vi "Pat 3.0.vi"(8 "error in":errorcluster, 11 "Father of all uServices in":refnum<class "Father of all uServices.lvclass">) -> (0 "error out":errorcluster, 3 "Father of all uServices out":refnum<class "Father of all uServices.lvclass">)   [LabVIEW 2026, in "TALOS.lvlib" / "Father of all uServices.lvlib" / "Father of all uServices.lvclass"]
uses:
  Father of all uServices.lvclass
  C:/LabVIEW Code/TALOS/talos/Ancestor/Ancestor/Ancestor.lvclass
  Ancestor/Ancestor/Ancestor.lvclass/Ancestor.ctl
  Classes/uService List/uService List.lvclass/uService List.ctl
  Classes/uService List/Set Last Pat.vi
  Classes/uService List/Set Online Status.vi
  Ancestor/Ancestor/Read ID.vi
  Ancestor/Ancestor/Write uS List Ref.vi
  Support VIs/Generate Error.vi
  FGV/Error Memory/Get Error Description.vi
  Support VIs/Get PC name.vi
  Support VIs/Get Class Name.vi
  <vilib>/Utility/error.llb/Clear Errors.vi
  FGV/Error Memory/Error Memory Core.vi
  <vilib>/AdvancedString/Delimited String to 1D String Array.vi
  <vilib>/AdvancedString/Delimited String to 1D String Array (string).vi
  Support VIs/Circus Root Path.vi
  FGV/Error Memory/Error Crt Lvl checker.vi
  FGV/Error Memory/Error Memory Core.vi/40c8088d-b597-4017-91af-faa98e00292e.vi
  FGV/Error Memory/Error Memory Core.vi/d4a3ab98-063c-4e44-b43d-fbdcfe6c2be2.vi
  Support VIs/Global Memory.vi
  <vilib>/Utility/LVClass/Get LV Class Name.vi
  Support VIs/Is in Packed Library.vi
  Support VIs/TALOS Root path.vi
  Support VIs/Read CSV worksheet.vi
  Support VIs/Global Constants.vi
  <vilib>/Utility/error.llb/General Error Handler.vi
  Support VIs/Error Log.vi
  Classes/uService List/uService List.lvclass
  Ancestor/Ancestor/Ancestor.lvclass
  <vilib>/Comparison/Equal/Equal Functor/Equal Functor.lvclass
  TALOS.lvlib
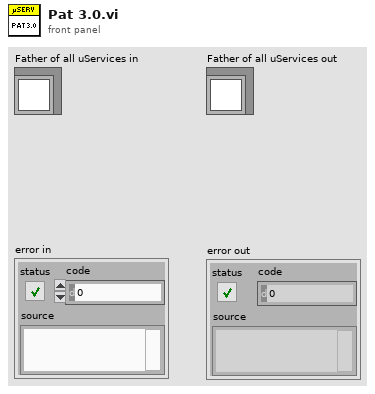
[diagram p1: front panel]
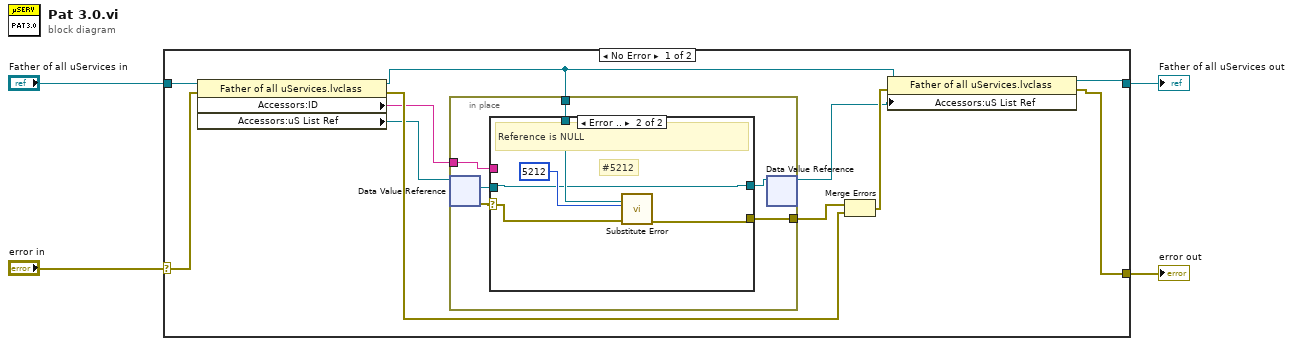
[diagram p0: block diagram]
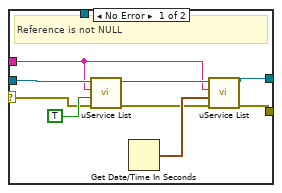
[diagram p2: hidden frame]
diagram:
  n1 = case shown="No Error" "error in" {
    selector: "error in" -> [w14 w36]
    tunnel: "Father of all uServices in" -> [w15 w37]
    tunnel: [w11 w36] -> w2
    tunnel: [w12 w37] -> w1
    frame No Error {
      n2 = property class="Father of all uServices.lvclass"(reference=w15, error in=w14) -> (reference out=w6:refnum<class "Father of all uServices.lvclass">, error out=w10:errorcluster, "Accessors:ID"=w9:string, "Accessors:uS List Ref"=w8:refnum<data-value>)
      n3 = in-place {
        in-place-border: w9 -> [w20]
        in-place-border: [w19] -> w5
        in-place-border: w6 -> [w16]
        n4 = in-place-dvr #1(w8) -> (w21:refnum<class "uService List.lvclass">, w17:errorcluster)
        n5 = case shown="Error .." w17 {
          selector: w17 -> [w22 w34]
          tunnel: w21 -> [w26 w31]
          tunnel: w20 -> [w25 _]
          tunnel: [w24 w32] -> w19
          tunnel: [w23 w31] -> w18
          tunnel: w16 -> [_ w33]
          frame No Error {
            # "Reference is not NULL"
            n6 = call-poly "uService List.vi"("error in (no error)"=w22, "Online"=TRUE, "ID"=w25, "uService List in"=w26) -> ("error out"=w27:errorcluster, "uService List out"=w28:refnum<class "uService List.lvclass">)  [unwired: 6 in]
            n7 = Get Date/Time In Seconds() -> (seconds since 1Jan1904=w30:timestamp)
            n8 = call-poly "uService List.vi"("error in (no error)"=w27, "Last Pat"=w30, "ID"=w25, "uService List in"=w28) -> ("error out"=w24:errorcluster, "uService List out"=w23:refnum<class "uService List.lvclass">)  [unwired: 6 in]
          }
          frame Error {
            # "#5212"
            # "Reference is NULL"
            n9 = call "Substitute Error.vi"("LabVIEW Object"=w33, "error in (no error)"=w34, "Error Code"=5212) -> ("error out"=w32:errorcluster)  [unwired: 8 in]
          }
        }
        n10 = in-place-dvr #1(w18) -> (w7:refnum<data-value>)  [unwired: 1 out]
      }
      n11 = Merge Errors(w5, w10) -> (w13:errorcluster)
      n12 = property class="Father of all uServices.lvclass"(reference=w6, error in=w13, "Accessors:uS List Ref"=w7) -> (reference out=w12:refnum<class "Father of all uServices.lvclass">, error out=w11:errorcluster)
    }
    frame Error {
    }
  }
  "error out" <- w2
  "Father of all uServices out" <- w1
